vi "RT Main.vi"() -> ()   [LabVIEW 2013]
doc: "This template is for the Queued Message Handler design pattern.\n\nThe Event Handling Loop generates messages based on user interface actions.\n\nThe Message Handling Loop processes messages generated by the Event Handling Loop, or by other messages. The messages are string values, so new messages can be added easily to the Message Cases case structure in the Message Handling Loop. Each message cluster can also provide an optional value for Message Data, which is a variant that can be converted to whatever message-specific data is required."
uses:
  <vilib>/userdefined/High Color/nirio_resource_hc.ctl
  controls/FPGA State.ctl
  controls/Raw Values.ctl
  controls/Control Configuration.ctl
  controls/Motion Observer.ctl
  controls/Digital Controller.ctl
  Globals/Global - All RT Loop Stop.vi
  Globals/Global - Configuration Options.vi
  <vilib>/rvi/errors/niLvFpgaAdjustHostInterfaceError.vi
  Globals/Global - RT Stream Connections.vi
  <vilib>/FPGAPlugInAG/cRIO-9075/niLvFpga_Close_cRIO-9075.vi
  <vilib>/rvi/interface/nirviReadWriteControl/nirviReadWriteControl.xnode
  controls/FPGA VI Reference.ctl
  FPGA Bitfiles/crio-FPGA-contro_FPGATarget_FPGAMain_4HKUk4gb9wY.lvbitx
  <vilib>/rvi/interface/nirviCloseFPGA/nirviCloseFPGA.xnode
  support/Message Queue/Message Queue.lvlib
  NiFpgaLv.dll
  <vilib>/nisyscfg/nisyscfg.lvlib
  <instrlib>/ZaberTSeries/ZaberTSeries.lvlib
panel:
  in  "VISA resource name":refnum<visa-resource-name>
  in  "cRIO resource name":T1
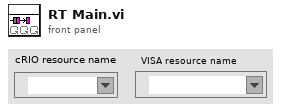
[diagram p1: front panel]
types:
  T1 = typedef "nirio_resource_hc.ctl" = tag
  T2 = typedef "FPGA VI Reference.ctl" = refnum<k20>
  T3 = typedef "FPGA State.ctl" = enum16{"Safe State", "Manual", "Control (PID)"}
  T4 = typedef "Control Configuration.ctl" = cluster{"PID Gains":cluster{"proportional gain (Kc)":fxp<+/-,16,8>, "integral gain (Kc*Ts/Ti)":fxp<+/-,16,8>, "derivative gain (Kc*Td/Ts)":fxp<+/-,16,8>}, "Output Range":cluster{"output high":fxp<+/-,16,7>, "output low":fxp<+/-,16,7>}}
  T5 = typedef "Digital Controller.ctl" = cluster{"kvc (N/m)":fxp<+,16,12>, "ymod (-)":fxp<+/-,16,5>, "Mar (kg)":fxp<+/-,16,8>, "Foff (N)":fxp<+/-,16,8>, "Fthresh (N)":fxp<+/-,16,5>, "ba (kg/s)":fxp<+/-,16,5>, "ksa (N/m)":fxp<+/-,16,5>, "kisa (N/m)":fxp<+/-,16,5>, "k_backemf":fxp<+/-,16,5>, "Frr (N/s)":fxp<+/-,16,5>, "xrr (mm/s)":fxp<+/-,16,5>, "bp (kg/s)":fxp<+/-,16,5>, "k_1 (1/s)":fxp<+/-,16,5>, "k_2 (1/s)":fxp<+/-,16,5>}
  T6 = typedef "Motion Observer.ctl" = cluster{"bo (kg/s)":fxp<+/-,20,7>, "kso (N/m)":fxp<+/-,20,7>, "kiso (N/m)":fxp<+/-,20,7>}
  T7 = typedef "Raw Values.ctl" = cluster{"Channel 0":fxp<+/-,20,7>, "Channel 1":fxp<+/-,20,7>, "Channel 2":fxp<+/-,20,7>, "Channel 3":fxp<+/-,20,14>}
  T8 = cluster{"Digital Controller":T5, "Motion Observer":T6}
  T9 = typedef "All FPGA Configuration Values.ctl" = cluster{"FPGA State":T3, "Manual Values":T7, "Setpoints":T7, "Control Configurations":T4[]}
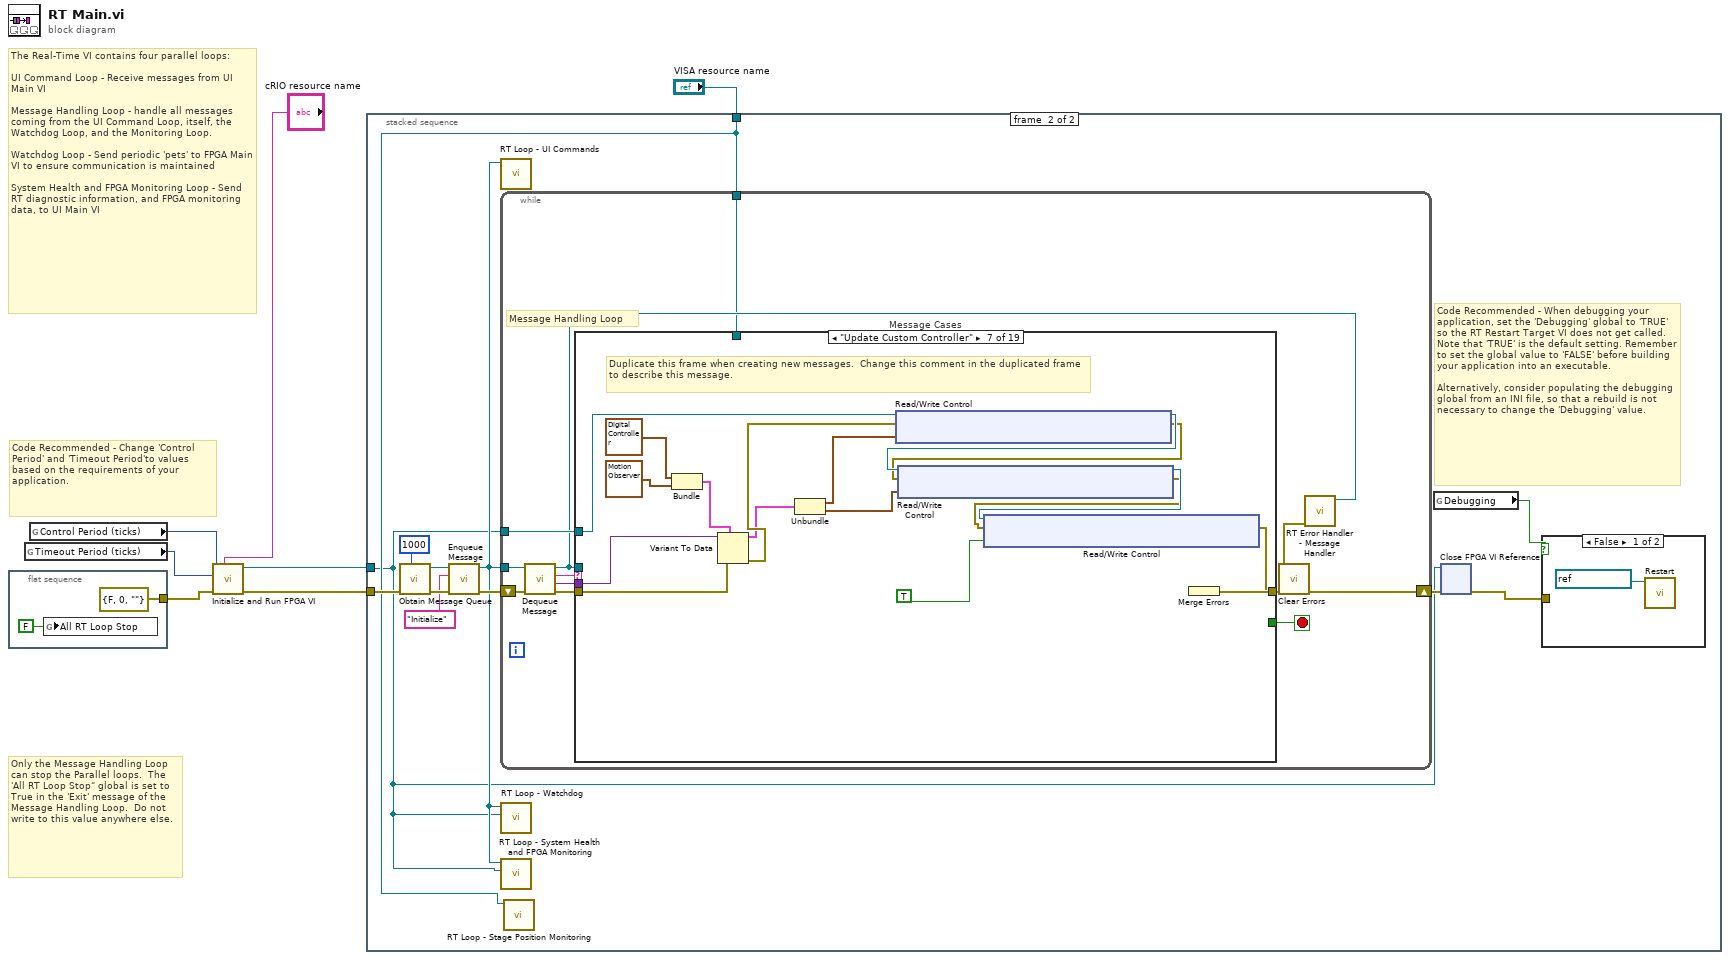
[diagram p0: block diagram]
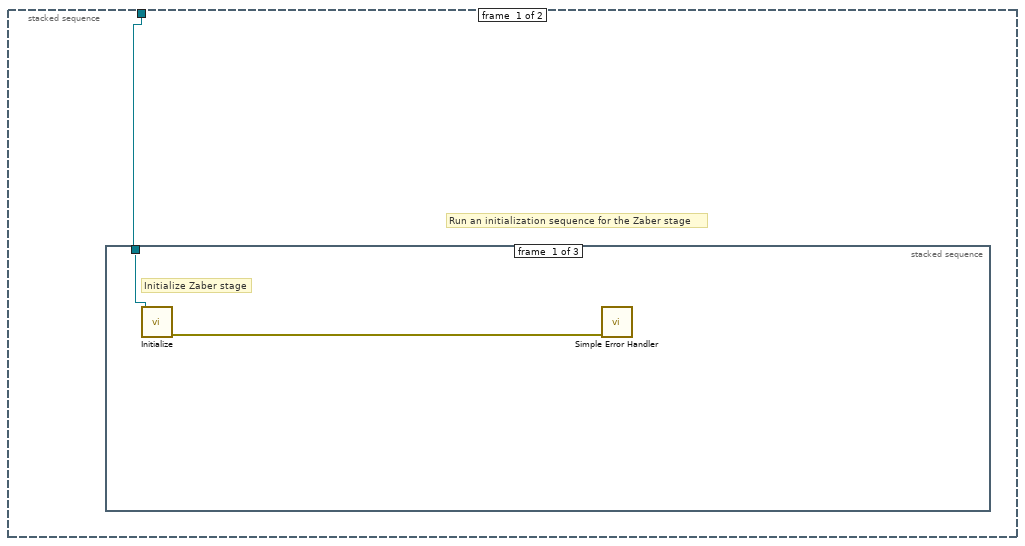
[diagram p2: hidden frame]
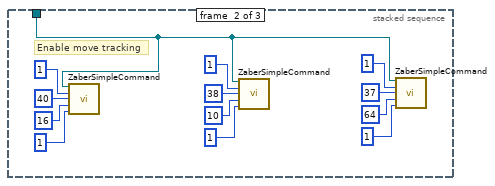
[diagram p3: hidden frame]
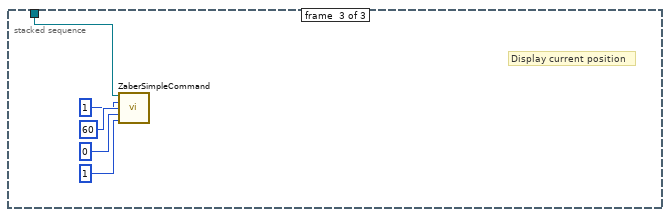
[diagram p4: hidden frame]
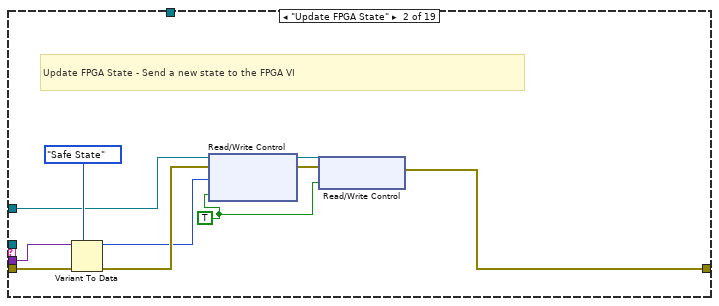
[diagram p7: hidden frame]
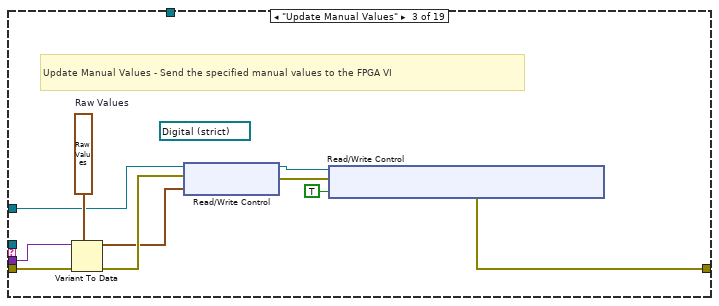
[diagram p8: hidden frame]
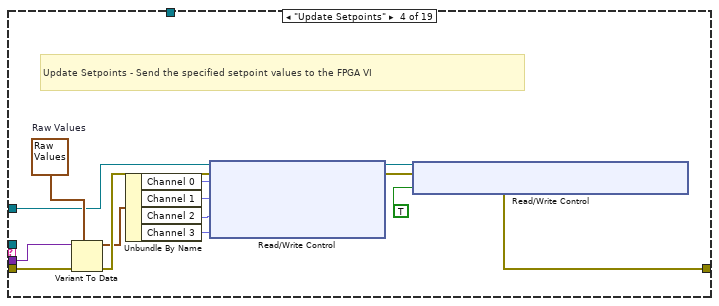
[diagram p9: hidden frame]
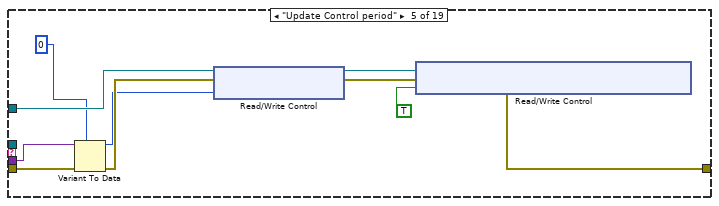
[diagram p10: hidden frame]
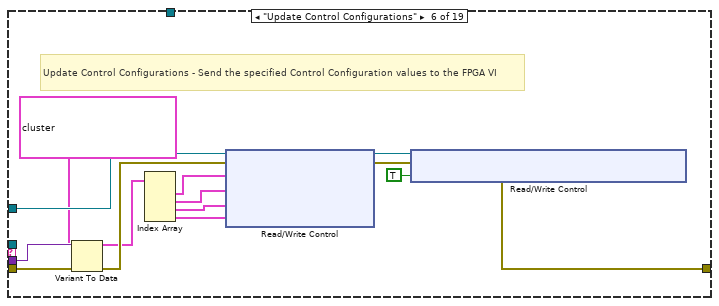
[diagram p11: hidden frame]
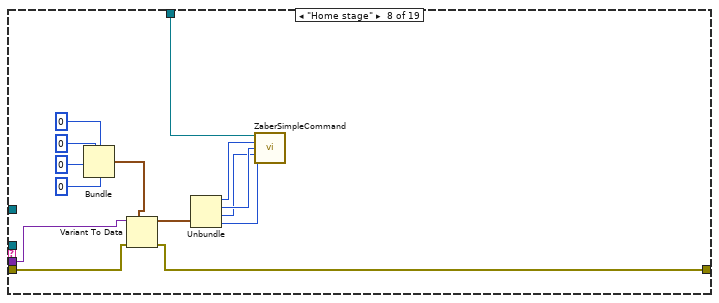
[diagram p12: hidden frame]
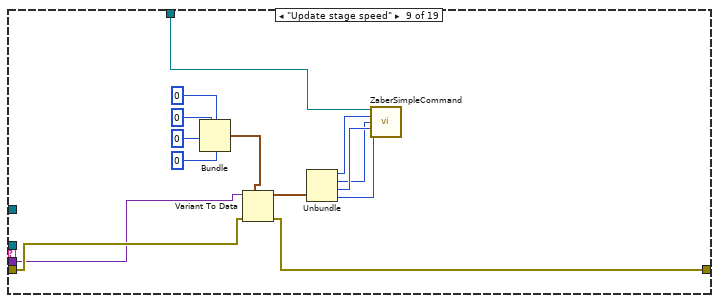
[diagram p13: hidden frame]
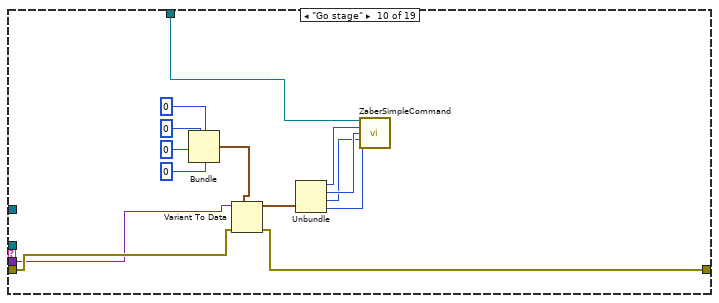
[diagram p14: hidden frame]
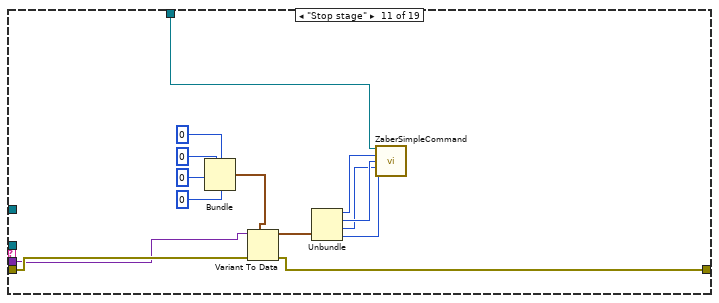
[diagram p15: hidden frame]
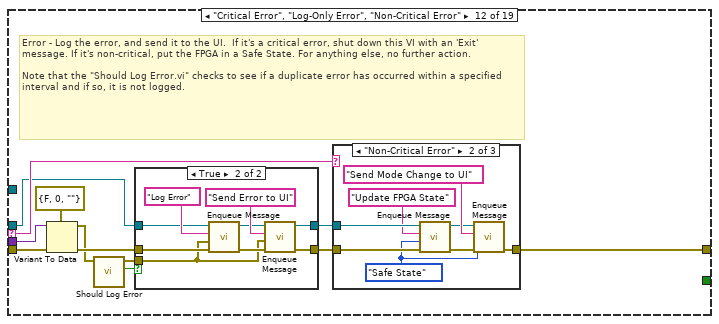
[diagram p16: hidden frame]
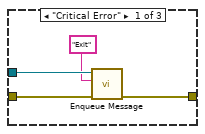
[diagram p18: hidden frame]
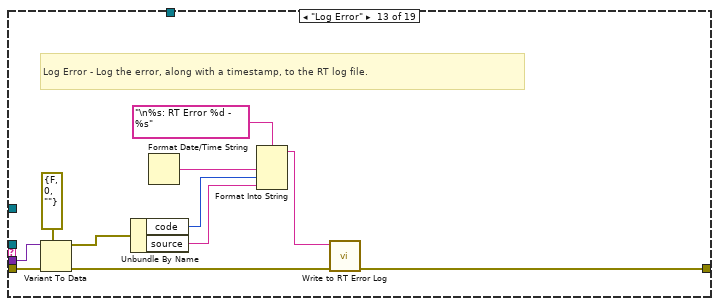
[diagram p20: hidden frame]
diagram:
  # "Code Recommended - Change 'Control Period' and 'Timeout Period'to values based on the requirements of your application."
  # "The Real-Time VI contains four parallel loops:\n\nUI Command Loop - Receive messages from UI Main VI\n\nMessage Handling Loop - handle all messages coming from the UI Command Loop, itself, the Watchdog Loop, and the Monitoring Loop.\n\nWatchdog Loop - Send periodic 'pets' to FPGA Main VI to ensure communication is maintained\n\nSystem Health and FPGA Monitoring Loop - Send RT diagnostic information, and FPGA monitoring data, to UI Main VI"
  # "Only the Message Handling Loop can stop the Parallel loops.  The 'All RT Loop Stop\" global is set to True in the 'Exit' message of the Message Handling Loop.  Do not write to this value anywhere else."
  n1 = flat-sequence {
    tunnel: [errorcluster {"status"=FALSE, "code"=0, "source"=""} ("error constant")] -> w6
    frame #0 {
      n2 = global write "Global - All RT Loop Stop.vi" "All RT Loop Stop"(FALSE) -> ()
    }
  }
  n3 = global read "Global - Configuration Options.vi" "Timeout Period (ticks)"() -> (w4:u64)
  n4 = global read "Global - Configuration Options.vi" "Control Period (ticks)"() -> (w5:u32)
  n5 = call "Initialize and Run FPGA VI.vi"("resource name"="cRIO resource name", "error in (no error)"=w6, "Timeout Period (ticks)"=w4, "Control Period (ticks)"=w5) -> ("error out"=w7:errorcluster, "FPGA VI Reference Out"=w3:T2)  [unwired: 6 in]
  n6 = stacked-sequence {
    tunnel: w7 -> [_ w33]
    tunnel: w3 -> [_ w31]
    tunnel: "VISA resource name" -> [w10 w32]
    frame #0 {
      # "Run an initialization sequence for the Zaber stage"
      n7 = stacked-sequence {
        tunnel: w10 -> [w11 w13 w26]
        frame #0 {
          # "Initialize Zaber stage"
          n8 = call <instrlib>:"Initialize.vi"("VISA resource name"=w11) -> ("error out"=w12:errorcluster)  [unwired: 8 in, 2 out]
          n9 = call <vilib>:"Simple Error Handler.vi"("error in (no error)"=w12) -> ()  [unwired: 4 in, 5 out]
        }
        frame #1 {
          # "Enable move tracking"
          n10 = call "ZaberSimpleCommand.vi"("VISA Refnum in"=w13, "Num1"=1, "Cmd"=40, "Val"=16, "Resp num"=1) -> ()  [unwired: 8 in, 3 out]
          n11 = call "ZaberSimpleCommand.vi"("VISA Refnum in"=w13, "Num1"=1, "Cmd"=38, "Val"=10, "Resp num"=1) -> ()  [unwired: 8 in, 3 out]
          n12 = call "ZaberSimpleCommand.vi"("VISA Refnum in"=w13, "Num1"=1, "Cmd"=37, "Val"=64, "Resp num"=1) -> ()  [unwired: 8 in, 3 out]
        }
        frame #2 {
          # "Display current position"
          n13 = call "ZaberSimpleCommand.vi"("VISA Refnum in"=w26, "Num1"=1, "Cmd"=60, "Val"=0, "Resp num"=1) -> ()  [unwired: 8 in, 3 out]
        }
      }
    }
    frame #1 {
      # "Code Recommended - When debugging your application, set the 'Debugging' global to 'TRUE' so the RT Restart Target VI does not get called.  Note that 'TRUE' is the default setting. Remember to set the global value to 'FALSE' before building your application into an executable.\n\nAlternatively, consider populating the debugging global from an INI file, so that a rebuild is not necessary to change the 'Debugging' value."
      n14 = call "Obtain Message Queue.vi"("max queue size (-1, unlimited)"=1000, "error in (no error)"=w33) -> ("error out"=w42:errorcluster, "Message Queue"=w41:refnum<queue>)  [unwired: 8 in]
      n15 = call "Enqueue Message.vi"("error in (no error)"=w42, "Message"="Initialize", "Message Queue"=w41) -> ("error out"=w39:errorcluster, "dup Message Queue"=w38:refnum<queue>)  [unwired: 7 in]
      n16 = call "RT Loop - UI Commands.vi"("Message Queue"=w38) -> ()  [unwired: 11 in]
      n17 = while {
        tunnel: w38 -> [w49]
        shift-right: [w46] -> w37
        shift-left: w39 -> [w53]
        tunnel: w31 -> [w48]
        tunnel: w32 -> [w44]
        stop <- w54 stop-if-true
        # "Message Handling Loop"
        n18 = call "Dequeue Message.vi"("error in (no error)"=w53, "Message Queue"=w49) -> ("error out"=w52:errorcluster, "Message Data"=w50:variant, "Message"=w51:string, "dup Message Queue"=w47:refnum<queue>)  [unwired: 6 in]
        n19 = case "Message Cases" shown="\"Update Custom Controller\"" w51 {
          selector: w51 -> [_ _ _ _ _ _ _ _ _ _ _ w196 _ _ _ _ _ _ w267]
          tunnel: w47 -> [_ _ _ _ _ _ _ _ _ _ _ w190 _ _ _ _ w261 _ _]
          tunnel: w52 -> [w55 w65 w75 w89 w94 w113 w129 w143 w148 w162 w176 w194 w233 w237 w243 w247 w257 w263 _]
          tunnel: [w55 w57 w66 w76 w95 w100 w130 w142 w145 w159 w175 w195 w224 w234 w238 w246 w258 w262 w265] -> w45
          tunnel: [_ _ _ _ _ _ _ _ _ _ _ _ _ _ _ _ TRUE _ _] -> w54
          tunnel: w50 -> [_ w64 w74 w88 w93 w112 w125 w141 w147 w161 w174 w193 w232 w236 _ w245 _ _ _]
          tunnel: w48 -> [_ w61 w71 w85 w92 w110 w128 _ _ _ _ _ _ _ w242 _ w253 _ _]
          tunnel: w44 -> [_ _ _ _ _ _ _ w144 w146 w160 w173 _ _ _ _ _ _ _ _]
          frame "Initialize" {
            # "Initialize - Currently a no-op for the RT Main VI"
          }
          frame "Update FPGA State" {
            w56 = TRUE ("Change State")
            # "Update FPGA State - Send a new state to the FPGA VI"
            n20 = Variant To Data(error in=w65, type=FPGA_State."Safe State" ("FPGA State"), Variant=w64) -> (data=w60:T3, error out=w62:errorcluster)
            n21 = xnode "Read/Write Control"("FPGA VI Reference In"=w61, "error in"=w62, "New State"=w60, "Change State"=w56) -> ("FPGA VI Reference Out"=w59:T2, "error out"=w58:errorcluster)
            n22 = xnode "Read/Write Control"("FPGA VI Reference In"=w59, "error in"=w58, "Disable Drive"=w56) -> ("error out"=w57:errorcluster)  [unwired: 1 out]
          }
          frame "Update Manual Values" {
            (unwired) refnum<vi> refnum ("Control period (ticks) Ref")
            w73 = T7 {"Channel 0"=0.0, "Channel 1"=0.0, "Channel 2"=0.0, "Channel 3"=0.0}  # Raw Values
            # "Update Manual Values - Send the specified manual values to the FPGA VI"
            n23 = Variant To Data(error in=w75, type=w73, Variant=w74) -> (data=w70:T7, error out=w72:errorcluster)
            n24 = xnode "Read/Write Control"("FPGA VI Reference In"=w71, "error in"=w72, "Manual Values"=w70) -> ("FPGA VI Reference Out"=w69:T2, "error out"=w68:errorcluster)
            n25 = xnode "Read/Write Control"("FPGA VI Reference In"=w69, "error in"=w68, "Enable Drive"=TRUE) -> ("error out"=w66:errorcluster)  [unwired: 1 out]
          }
          frame "Update Setpoints" {
            w87 = T7 {"Channel 0"=0.0, "Channel 1"=0.0, "Channel 2"=0.0, "Channel 3"=0.0}  # Raw Values
            # "Update Setpoints - Send the specified setpoint values to the FPGA VI"
            n26 = Variant To Data(error in=w89, type=w87, Variant=w88) -> (data=w84:T7, error out=w86:errorcluster)
            n27 = Unbundle By Name(w84) -> ("Channel 0"=w83:fxp<+/-,20,7>, "Channel 1"=w80:fxp<+/-,20,7>, "Channel 2"=w82:fxp<+/-,20,7>, "Channel 3"=w81:fxp<+/-,20,14>)
            n28 = xnode "Read/Write Control"("FPGA VI Reference In"=w85, "error in"=w86, "Channel 0 Setpoint (Force)"=w83, "Channel 1 Setpoint  (Position)"=w80, "Channel 2 Setpoint"=w82, "Channel 3 Setpoint"=w81) -> ("FPGA VI Reference Out"=w77:T2, "error out"=w78:errorcluster)
            n29 = xnode "Read/Write Control"("FPGA VI Reference In"=w77, "error in"=w78, "Enable Drive"=TRUE) -> ("error out"=w76:errorcluster)  [unwired: 1 out]
          }
          frame "Update Control period" {
            n30 = Variant To Data(error in=w94, type=u32 0 ("Control period (ticks)"), Variant=w93) -> (data=w90:u32, error out=w96:errorcluster)
            n31 = xnode "Read/Write Control"("FPGA VI Reference In"=w92, "error in"=w96, "Control Period (ticks)"=w90) -> ("FPGA VI Reference Out"=w99:T2, "error out"=w98:errorcluster)
            n32 = xnode "Read/Write Control"("FPGA VI Reference In"=w99, "error in"=w98, "Enable Drive"=TRUE) -> ("error out"=w95:errorcluster)  [unwired: 1 out]
          }
          frame "Update Control Configurations" {
            # "Update Control Configurations - Send the specified Control Configuration values to the FPGA VI"
            n33 = Variant To Data(error in=w113, type=T4[] [{"PID Gains"={"proportional gain (Kc)"=0.0, "integral gain (Kc*Ts/Ti)"=0.0, "derivative gain (Kc*Td/Ts)"=0.0}, "Output Range"={"output high"=0.0, "output low"=0.0}}], Variant=w112) -> (data=w108:T4[], error out=w111:errorcluster)
            n34 = Index Array(array=w108) -> (element #1=w107:T4, element #2=w106:T4, element #3=w105:T4, element #4=w104:T4)  [unwired: 4 in]
            n35 = xnode "Read/Write Control"("FPGA VI Reference In"=w110, "error in"=w111, "Channel 0 Configuration"=w107, "Channel 1 Configuration"=w106, "Channel 2 Configuration"=w105, "Channel 3 Configuration"=w104) -> ("FPGA VI Reference Out"=w102:T2, "error out"=w101:errorcluster)
            n36 = xnode "Read/Write Control"("FPGA VI Reference In"=w102, "error in"=w101, "Enable Drive"=TRUE) -> ("error out"=w100:errorcluster)  [unwired: 1 out]
          }
          frame "Update Custom Controller" {
            # "Duplicate this frame when creating new messages.  Change this comment in the duplicated frame to describe this message."
            n37 = Bundle("Digital Controller"=T5 {"kvc (N/m)"=0.0, "ymod (-)"=0.0, "Mar (kg)"=0.0, "Foff (N)"=0.1640625, "Fthresh (N)"=0.0, "ba (kg/s)"=0.0, "ksa (N/m)"=0.0, "kisa (N/m)"=0.0, "k_backemf"=0.0, "Frr (N/s)"=0.0, "xrr (mm/s)"=0.0, "bp (kg/s)"=0.0, "k_1 (1/s)"=0.0, "k_2 (1/s)"=0.0}, "Motion Observer"=T6 {"bo (kg/s)"=0.0, "kso (N/m)"=0.0, "kiso (N/m)"=0.0}) -> (w121:T8)  [unwired: 1 in]
            n38 = Variant To Data(error in=w129, type=w121, Variant=w125) -> (data=w120:T8, error out=w124:errorcluster)
            n39 = Unbundle(w120) -> ("Digital Controller"=w119:T5, "Motion Observer"=w116:T6)
            n40 = xnode "Read/Write Control"("FPGA VI Reference In"=w128, "error in"=w124, "Digital Controller"=w119) -> ("FPGA VI Reference Out"=w118:T2, "error out"=w117:errorcluster)
            n41 = xnode "Read/Write Control"("FPGA VI Reference In"=w118, "error in"=w117, "Motion Observer"=w116) -> ("FPGA VI Reference Out"=w115:T2, "error out"=w114:errorcluster)
            n42 = xnode "Read/Write Control"("FPGA VI Reference In"=w115, "error in"=w114, "Enable Drive"=TRUE) -> ("error out"=w126:errorcluster)  [unwired: 1 out]
            n43 = Merge Errors(w126) -> (w130:errorcluster)
          }
          frame "Home stage" {
            n44 = Bundle(0, 0, 0, 0) -> (w136:cluster{i32, i32, i32, i32})  [unwired: 1 in]
            n45 = Variant To Data(error in=w143, type=w136, Variant=w141) -> (data=w135:cluster{i32, i32, i32, i32}, error out=w142:errorcluster)
            n46 = Unbundle(w135) -> (w134:i32, w133:i32, w132:i32, w131:i32)
            n47 = call "ZaberSimpleCommand.vi"("VISA Refnum in"=w144, "Num1"=w134, "Cmd"=w133, "Val"=w132, "Resp num"=w131) -> ()  [unwired: 8 in, 3 out]
          }
          frame "Update stage speed" {
            n48 = Bundle(0, 0, 0, 0) -> (w153:cluster{i32, i32, i32, i32})  [unwired: 1 in]
            n49 = Variant To Data(error in=w148, type=w153, Variant=w147) -> (data=w154:cluster{i32, i32, i32, i32}, error out=w145:errorcluster)
            n50 = Unbundle(w154) -> (w155:i32, w156:i32, w157:i32, w158:i32)
            n51 = call "ZaberSimpleCommand.vi"("VISA Refnum in"=w146, "Num1"=w155, "Cmd"=w156, "Val"=w157, "Resp num"=w158) -> ()  [unwired: 8 in, 3 out]
          }
          frame "Go stage" {
            n52 = Bundle(0, 0, 0, 0) -> (w168:cluster{i32, i32, i32, i32})  [unwired: 1 in]
            n53 = Variant To Data(error in=w162, type=w168, Variant=w161) -> (data=w167:cluster{i32, i32, i32, i32}, error out=w159:errorcluster)
            n54 = Unbundle(w167) -> (w166:i32, w165:i32, w164:i32, w163:i32)
            n55 = call "ZaberSimpleCommand.vi"("VISA Refnum in"=w160, "Num1"=w166, "Cmd"=w165, "Val"=w164, "Resp num"=w163) -> ()  [unwired: 8 in, 3 out]
          }
          frame "Stop stage" {
            n56 = Bundle(0, 0, 0, 0) -> (w182:cluster{i32, i32, i32, i32})  [unwired: 1 in]
            n57 = Variant To Data(error in=w176, type=w182, Variant=w174) -> (data=w181:cluster{i32, i32, i32, i32}, error out=w175:errorcluster)
            n58 = Unbundle(w181) -> (w180:i32, w179:i32, w178:i32, w177:i32)
            n59 = call "ZaberSimpleCommand.vi"("VISA Refnum in"=w173, "Num1"=w180, "Cmd"=w179, "Val"=w178, "Resp num"=w177) -> ()  [unwired: 8 in, 3 out]
          }
          frame "Critical Error", "Log-Only Error", "Non-Critical Error" {
            # "Error - Log the error, and send it to the UI.  If it's a critical error, shut down this VI with an 'Exit' message. If it's non-critical, put the FPGA in a Safe State. For anything else, no further action.\n\nNote that the \"Should Log Error.vi\" checks to see if a duplicate error has occurred within a specified interval and if so, it is not logged."
            n60 = Variant To Data(error in=w194, type=errorcluster {"status"=FALSE, "code"=0, "source"=""} ("error out"), Variant=w193) -> (data=w188:errorcluster, error out=w191:errorcluster)
            n61 = call "Should Log Error.vi"("error to report"=w188) -> ("Should Log Error?"=w189:bool, "dup error to report"=w187:errorcluster)  [unwired: 9 in]
            n62 = case shown="True" w189 {
              tunnel: [w200 w207] -> w198
              tunnel: [w199 w206] -> w197
              tunnel: w190 -> [w199 w205]
              tunnel: w191 -> [w200 w202]
              tunnel: w187 -> [_ w201]
              frame False {
              }
              frame True {
                n63 = call "Enqueue Message.vi"("error in (no error)"=w202, "Message Data"=w201, "Message"="Log Error", "Message Queue"=w205) -> ("error out"=w203:errorcluster, "dup Message Queue"=w204:refnum<queue>)  [unwired: 6 in]
                n64 = call "Enqueue Message.vi"("error in (no error)"=w203, "Message Data"=w201, "Message"="Send Error to UI", "Message Queue"=w204) -> ("error out"=w207:errorcluster, "dup Message Queue"=w206:refnum<queue>)  [unwired: 6 in]
              }
            }
            n65 = case shown="\"Non-Critical Error\"" w196 {
              tunnel: w198 -> [w213 w221 w222]
              tunnel: w197 -> [w211 w220 _]
              tunnel: [w212 w217 w222] -> w195
              frame "Critical Error" {
                n66 = call "Enqueue Message.vi"("error in (no error)"=w213, "Message"="Exit", "Message Queue"=w211) -> ("error out"=w212:errorcluster)  [unwired: 7 in, 1 out]
              }
              frame "Non-Critical Error" {
                w214 = FPGA_State."Safe State" ("FPGA State")
                n67 = call "Enqueue Message.vi"("error in (no error)"=w221, "Message Data"=w214, "Message"="Update FPGA State", "Message Queue"=w220) -> ("error out"=w218:errorcluster, "dup Message Queue"=w215:refnum<queue>)  [unwired: 6 in]
                n68 = call "Enqueue Message.vi"("error in (no error)"=w218, "Message Data"=w214, "Message"="Send Mode Change to UI", "Message Queue"=w215) -> ("error out"=w217:errorcluster)  [unwired: 6 in, 1 out]
              }
              frame Default {
              }
            }
          }
          frame "Log Error" {
            # "Log Error - Log the error, along with a timestamp, to the RT log file."
            n69 = Variant To Data(error in=w233, type=errorcluster {"status"=FALSE, "code"=0, "source"=""} ("error constant"), Variant=w232) -> (data=w227:errorcluster, error out=w230:errorcluster)
            n70 = Unbundle By Name(w227) -> ("code"=w226:i32, "source"=w225:string)
            n71 = Format Date/Time String() -> (date/time string=w228:string)  [unwired: 3 in]
            n72 = Format Into String(format string="\n%s: RT Error %d - %s", w228, w226, w225) -> (resulting string=w223:string)  [unwired: 2 in, 1 out]
            n73 = call "Write to RT Error Log.vi"("error in (no error)"=w230, "Log Entry"=w223) -> ("error out"=w224:errorcluster)  [unwired: 9 in]
          }
          frame "Send Error to UI" {
            # "Send Error to UI - Send the error message to the UI. Ignore if a stream has not been established."
            n74 = call "RT - Send Message to UI.vi"("error in (no error)"=w237, "Message Data"=w236, "Message"="RT Error") -> ("error out"=w234:errorcluster)  [unwired: 8 in]
          }
          frame "Send FPGA Configuration to UI" {
            # "Send FPGA Configuration to UI - Send all FPGA configuration values to the UI. Ignore if a stream has not been established."
            n75 = call "Bundle FPGA Configuration.vi"("error in (no error)"=w243, "FPGA Interface (Old)"=w242) -> ("error out"=w241:errorcluster, "All FPGA Configuration Values"=w240:T9)  [unwired: 8 in]
            n76 = call "RT - Send Message to UI.vi"("error in (no error)"=w241, "Message Data"=w240, "Message"="Initial UI Values") -> ("error out"=w238:errorcluster)  [unwired: 8 in]
          }
          frame "Send Mode Change to UI" {
            # "Send Mode Change to UI - Let the UI Main VI know that the mode of the FPGA Main VI has changed."
            n77 = call "RT - Send Message to UI.vi"("error in (no error)"=w247, "Message Data"=w245, "Message"="Update Display Mode") -> ("error out"=w246:errorcluster)  [unwired: 8 in]
          }
          frame "Exit" {
            # "Flush the Writer Stream to ensure all pending messages are sent to UI Main VI"
            # "Destroy streams on exit"
            # "Put FPGA VI in a Safe State on Exit"
            # "Stop Message Handling Loop"
            # "Stop All Parallel Loops"
            # "Release the message queue reference"
            n78 = global read "Global - RT Stream Connections.vi" "RT Writer Stream"() -> (w250:refnum<k21>)
            n79 = global read "Global - RT Stream Connections.vi" "UI Writer Stream"() -> (w252:refnum<k21>)
            n80 = Flush Stream(11:w250) -> (0:w248:errorcluster, 3:w249:refnum<k21>)  [unwired: 3 in, 1 out]
            n81 = Release Queue(queue=w261, error in (no error)=w257) -> (error out=w259:errorcluster)  [unwired: 1 in, 2 out]
            n82 = Destroy Stream Endpoint(8:w248, 11:w249) -> (0:w251:errorcluster)
            n83 = Destroy Stream Endpoint(8:w251, 11:w252) -> ()  [unwired: 1 out]
            n84 = xnode "Read/Write Control"("FPGA VI Reference In"=w253, "New State"=FPGA_State."Safe State", "Change State"=TRUE) -> ()  [unwired: 1 in, 2 out]
            n85 = global write "Global - All RT Loop Stop.vi" "All RT Loop Stop"(TRUE ("Stop Monitoring Loops")) -> ()
            n86 = Merge Errors(w259) -> (w258:errorcluster)
          }
          frame "---Copy This Frame---" {
            # "Duplicate this frame when creating new messages.  Change this comment in the duplicated frame to describe this message."
            n87 = Merge Errors(w263) -> (w262:errorcluster)
          }
          frame Default {
            # "'Default' case only runs if there is a message that isn't defined in any of the other cases.  Output a programming error."
            n88 = Format Into String(format string="The invalid message string \"%s\" was received in the Message Handling Loop." ("Unknown Message Error Text"), w267) -> (resulting string=w264:string)  [unwired: 2 in, 1 out]
            n89 = call <vilib>:"Error Cluster From Error Code.vi"("error message (\"\")"=w264, "error code (0)"=1) -> ("error out"=w265:errorcluster)  [unwired: 7 in]
          }
        }
        n90 = call <vilib>:"Clear Errors.vi"("error in (no error)"=w45) -> ("error out"=w46:errorcluster)  [unwired: 6 in]
        n91 = call "RT Error Handler - Message Handler.vi"("error in (no error)"=w45, "Message Queue"=w47) -> ()  [unwired: 9 in, 1 out]
      }
      n92 = call "RT Loop - Watchdog.vi"("FPGA VI Reference Out"=w31, "Message Queue"=w38) -> ()  [unwired: 10 in]
      n93 = call "RT Loop - System Health and FPGA Monitoring.vi"("FPGA VI Reference Out"=w31, "Message Queue"=w38) -> ()  [unwired: 10 in]
      n94 = call "RT Loop - Stage Position Monitoring.vi"("VISA resource name"=w32) -> ()  [unwired: 11 in]
      n95 = global read "Global - Configuration Options.vi" "Debugging"() -> (w35:bool)
      n96 = xnode "Close FPGA VI Reference"("FPGA VI Reference In"=w31, "error in"=w37) -> ("error out"=w36:errorcluster)
      n97 = case shown="False" w35 {
        tunnel: w36 -> [_ _]
        frame False {
          n98 = call <vilib>:"Restart.vi"("session in"=refnum<k21> "localhost") -> ()  [unwired: 8 in, 3 out]
        }
        frame True {
        }
      }
    }
  }
